vi "Get Key Value.vi"(8 "error in (no error)":errorcluster, 10 "Key":string, 11 "YAML Parser in":refnum<class "YAML Parser.lvclass">) -> (0 "error out":errorcluster, 1 "Is Null?":bool, 2 "Key Value":variant, 3 "YAML Parser out":refnum<class "YAML Parser.lvclass">)   [LabVIEW 2015, in "YAML Parser.lvclass"]
uses:
  YAML Parser.lvclass
  YAML Parser.lvclass/YAML Parser.ctl
  <vilib>/Utility/error.llb/Error Cluster From Error Code.vi
  <vilib>/ErrorRing/Error Ring.xnode
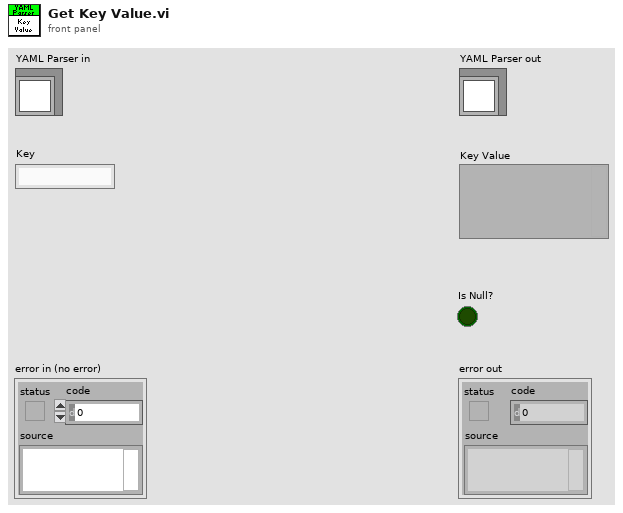
[diagram p1: front panel]
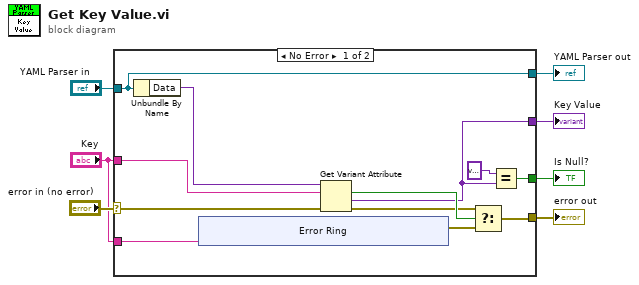
[diagram p0: block diagram]
diagram:
  n1 = case shown="No Error" "error in (no error)" {
    selector: "error in (no error)" -> [w17 w28]
    tunnel: [w11 w28] -> w6
    tunnel: [w18 w27] -> w4
    tunnel: "YAML Parser in" -> [w18 w27]
    tunnel: "Key" -> [w16 _]
    tunnel: "Key" -> [w15 _]
    tunnel: [w9 _] -> w2
    tunnel: [w8 _] -> w1
    frame No Error {
      n2 = Unbundle By Name(w18) -> ("Data"=w19:variant)
      n3 = xnode "Error Ring"("parameter 0"=w15) -> ("error out"=w12:errorcluster)
      n4 = Get Variant Attribute(Variant=w19, name=w16, error in=w17) -> (found=w14:bool, value=w9:variant, error out=w13:errorcluster)  [unwired: 1 in, 1 out]
      n5 = Select(t=w13, s=w14, f=w12) -> (s? t:f=w11:errorcluster)
      n6 = Equal?(x=variant, y=w9) -> (x = y?=w8:bool)
    }
    frame Error {
    }
  }
  "error out" <- w6
  "YAML Parser out" <- w4
  "Key Value" <- w2
  "Is Null?" <- w1
